vi "AM.vi"() -> ()   [LabVIEW 2018]
uses:
  <vilib>/express/express analysis/Spectral/Block/exnSpectralBlock spectral measurements peak poly.vi
  <vilib>/express/express analysis/Spectral/Block/exnSpectralBlock spectral measurements peak WFM.vi
  <vilib>/express/express analysis/Spectral/XNode/ExpressSpectralMeasurementsBlockNode.xnode
  <vilib>/measure/NI_MABase.lvlib
panel:
  in  "直流分量":dbl
  out "AM信号频谱":cluster{"f0":dbl, "df":dbl, "magnitude":dbl[]}(graph)
  out "AM检波信号":dynamicdata(graph)
  out "AM信号":waveform(dbl)(graph)
  out "基带频率":cluster{"f0":dbl, "df":dbl, "magnitude":dbl[]}(graph)
  out "基带信号":waveform(dbl)(graph)
  in  "载波幅度":dbl
  in  "载波频率":dbl
  in  "基带幅度":dbl
  in  "基带频率":dbl
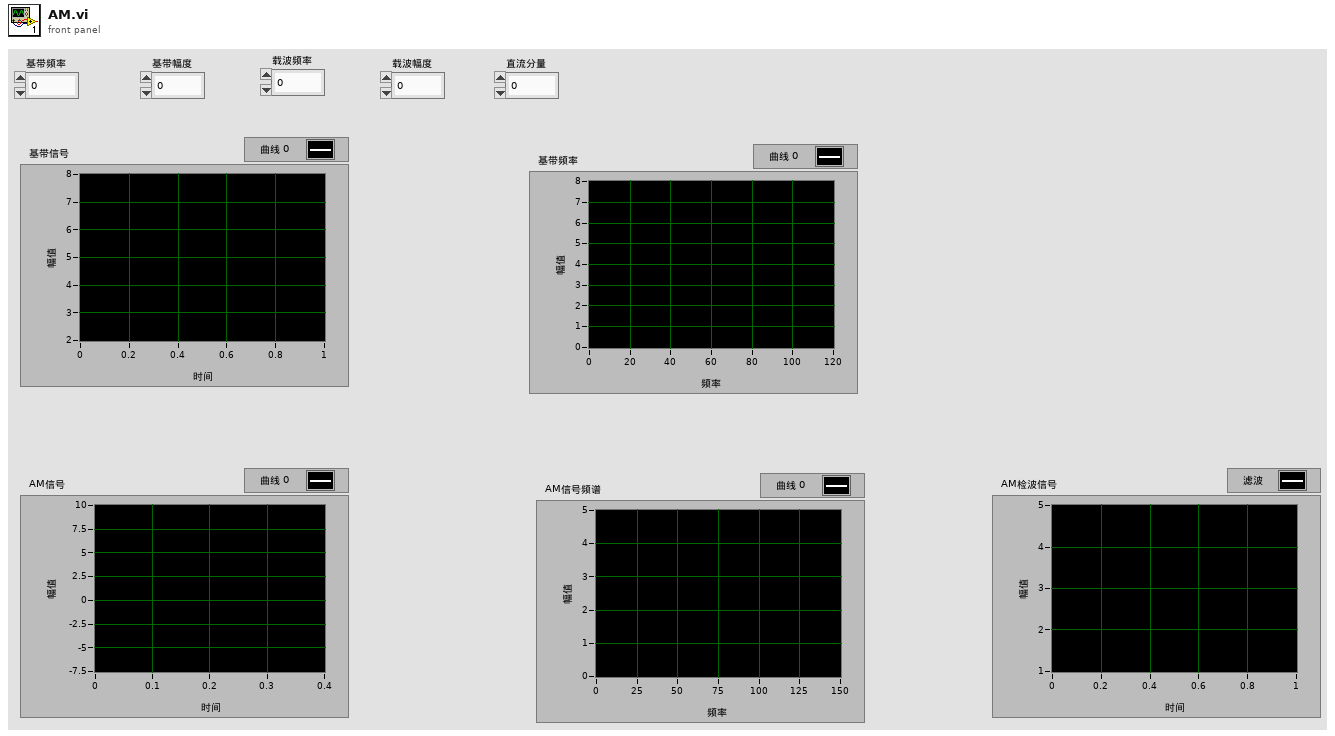
[diagram p1: front panel]
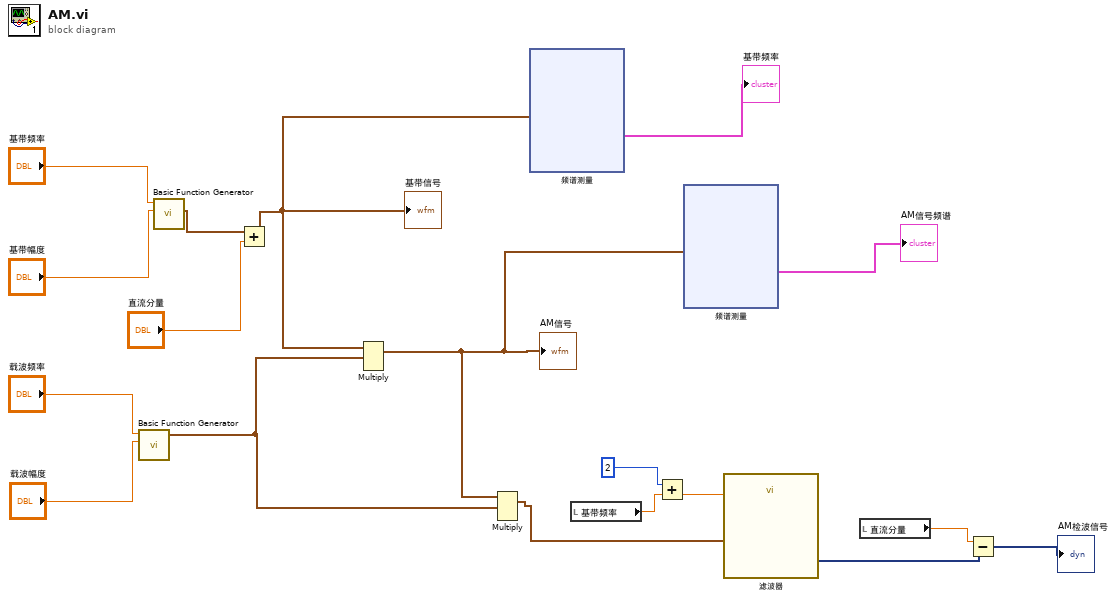
[diagram p0: block diagram]
diagram:
  n1 = call <vilib>:"Basic Function Generator.vi"("amplitude"="载波幅度", "frequency"="载波频率") -> ("signal out"=w4:waveform(dbl))  [unwired: 7 in, 2 out]
  n2 = call <vilib>:"Basic Function Generator.vi"("amplitude"="基带幅度", "frequency"="基带频率") -> ("signal out"=w6:waveform(dbl))  [unwired: 7 in, 2 out]
  n3 = Add(x=w6, y="直流分量") -> (x+y=w5:waveform(dbl))
  "基带信号" <- w5
  n4 = Multiply(1:w4, 2:w5) -> (0:w9:waveform(dbl))  [unwired: 1 in, 1 out]
  "AM信号" <- w9
  n5 = Multiply(1:w4, 2:w9) -> (0:w11:waveform(dbl))  [unwired: 1 in, 1 out]
  n6 = xnode "频谱测量"("信号"=w5) -> ("FFT - （峰值）"=→"基带频率":cluster{"f0":dbl, "df":dbl, "magnitude":dbl[]})  [unwired: 1 in, 2 out]
  n7 = local read "基带频率"() -> (w12:dbl)
  n8 = Add(x=2, y=w12) -> (x+y=w14:dbl)
  n9 = xnode "频谱测量"("信号"=w9) -> ("FFT - （峰值）"=→"AM信号频谱":cluster{"f0":dbl, "df":dbl, "magnitude":dbl[]})  [unwired: 1 in, 2 out]
  n10 = call "滤波器"("Lower Cut-Off"=w14, "Signal"=w11) -> ("Filtered Signal"=w3:dynamicdata)  [unwired: 8 in, 1 out]
  n11 = local read "直流分量"() -> (w2:dbl)
  n12 = Subtract(x=w2, y=w3) -> (x-y=→"AM检波信号":dynamicdata)
